vi "Global_CMD_Data Out.vi"() -> ()   [LabVIEW 2020, in "2023-Auto_CMD.lvlib"]
uses:
  2023-Auto_CMD.lvlib
  ENUM_CMD_State.ctl
  ENUM_Drive Mode Select.ctl
  Shared Code/TypeDefs/ENUM_Grabber_CMD_Mode Select.ctl
  MotionMaser/ENUM_Pose List.ctl
  MotionMaser/MotionMaster_SubCMD.lvlib
  Shared Code/TypeDefs/Dial_Compase heading unit circle CCW positive.ctl
  Shared Code/TypeDefs/Cluster_Auto Sequence Settings.ctl
  Shared Code/TypeDefs/Cluster_Auto Sequence Data.ctl
panel:
  in  "Single Step":T1={"State"=enum."Starting", "Max Wait Time (S)"=0.0, "CMDs"={"Drive Mode"=enum."Coast", "Auto Angle"=0.0, "Auto Target (ft)"=0.0, "Max speed ft/s"=0.0, "Arm Pose "=enum."None-Unknown", "Grabber CMD"=enum."STOP"}, "Color Box"=16448250} caption="Current Step" {"CMDs"."Auto Angle" scale format="%.3f"}
  in  "CMD_Template_CycleTime(S)":dbl
  # "The Names of the Data items in the Global Variable MUST describe who the Single Writer is\nFor CMD Globals the the naming convention is\n   \nCMD_Lib Name_Data Name\n\nExamples:\nCMD_RobotArm_Mode\nCMD_AutoTrack_Mode"
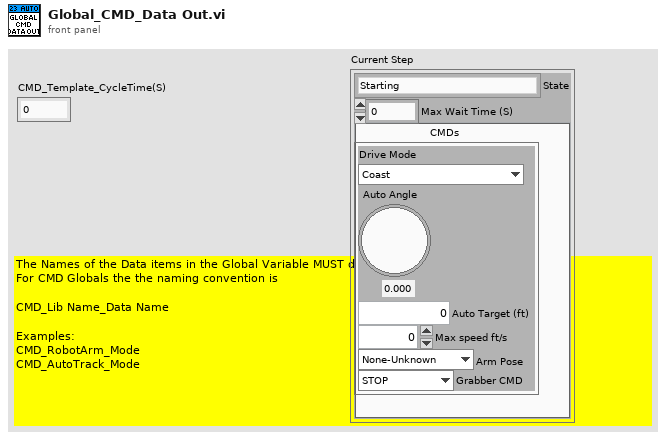
[diagram p1: front panel]
types:
  T1 = typedef "Cluster_Auto Sequence Data.ctl" = cluster{"State":T2, "Max Wait Time (S)":dbl, "CMDs":T3, "Color Box":u32}
  T2 = typedef "2023-Auto_CMD.lvlib/ENUM_CMD_State.ctl" = enum16{"Starting", "Idling", "Selecting Sequence", "Selecting Next Step", "Driving to Position", "Stopping", "Grabbing", "Moving Arm", "Rotation Target", "Waiting", "Shutting Down", "Balancing Level", "Configuring", "Tilt UP or Position", "Tile DOWN or Position", "LEVEL or Position"}
  T3 = typedef "Cluster_Auto Sequence Settings.ctl" = cluster{"Drive Mode":T4, "Auto Angle":T5, "Auto Target (ft)":dbl, "Max speed ft/s":dbl, "Arm Pose ":T6, "Grabber CMD":T7}
  T4 = typedef "2023-Auto_CMD.lvlib/ENUM_Drive Mode Select.ctl" = enum16{"Coast", "To Position", "Rotation Absolute", "Balance on Charger", "Brake", "Lock"}
  T5 = typedef "Dial_Compase heading unit circle CCW positive.ctl" = dbl
  T6 = typedef "MotionMaster_SubCMD.lvlib/ENUM_Pose List.ctl" = enum16{"None-Unknown", "Intake", "Score High", "Score Mid", "Safe Position", "Home Pos"}
  T7 = typedef "ENUM_Grabber_CMD_Mode Select.ctl" = enum16{"STOP", "Intake", "Eject"}
diagram:
